vi "Panel.vi"(11 "Dashboard Panel in":refnum<class "Dashboard Panel.lvclass">) -> ()   [LabVIEW 2020, in "SB App.lvlib" / "Dashboard Panel.lvclass"]
uses:
  Dashboard Panel.lvclass
  C:/Program Files (x86)/National Instruments/LabVIEW 2020/vi.lib/IlluminatedG/IG OOPanel/OOPanel/Panel/Panel.lvclass
  Sort Type.ctl
  <vilib>/IlluminatedG/IG OOPanel/OOPanel/Panel/Basic UI State.ctl
  Dashboard Panel.lvclass/Dashboard Panel.ctl
  Team Dashboard Panel/Team Dashboard Panel.lvclass
  C:/Program Files (x86)/National Instruments/LabVIEW 2020/vi.lib/IlluminatedG/IG OOPanel/OOPanel/ArrayPanel/ArrayPanel.lvclass
  Active Sort.vi
  Killed Sort.vi
  Attacked Sort.vi
  Collisions Sort.vi
  Replicated Sort.vi
  <vilib>/IlluminatedG/IG OOPanel/OOPanel/ArrayManager/ArrayManager.lvclass
  SquareBattle/Team/Team.lvclass
  <vilib>/IlluminatedG/IG OOPanel/OOPanel/Panel/Panel.lvclass
  <vilib>/IlluminatedG/IG OOPanel/OOPanel/OOPanel.lvlib
panel:
  in  "Sort":T1
  out "Round":u32
  in  "Stop":bool
  in  "Step":bool
  in  "Start":bool
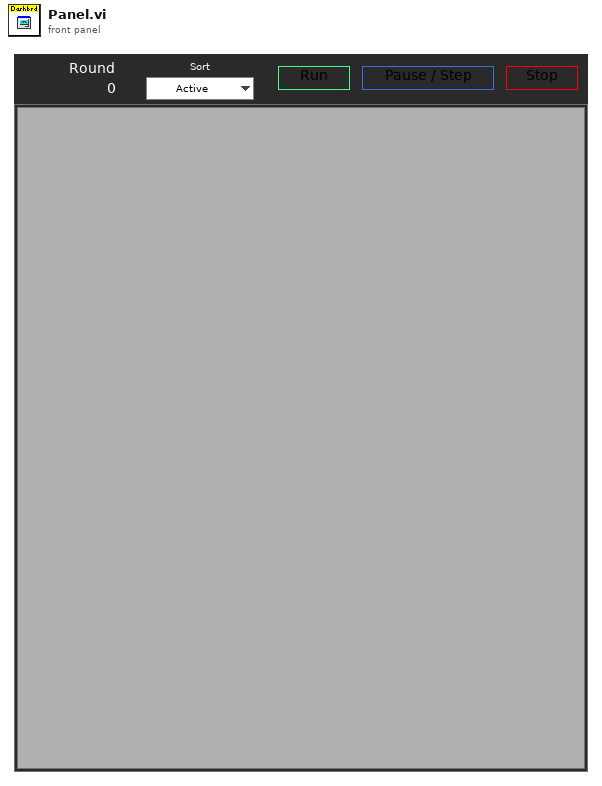
[diagram p1: front panel]
types:
  T1 = typedef "SB App.lvlib/Dashboard Panel.lvclass/Sort Type.ctl" = enum16{"Active", "Kills", "Attacked", "Collisions", "Replications"}
  T2 = typedef "OOPanel.lvlib/Panel.lvclass/Basic UI State.ctl" = enum16{"Init", "Run", "Close"}
  T3 = enum8{"Enabled", "Disabled", "Disabled and Grayed Out"}
  T4 = typedef "SB App.lvlib/Dashboard Panel.lvclass/Incoming Events.ctl" = cluster{"Round":refnum<user-event>, "Teams":refnum<user-event>, "Team Stats":refnum<user-event>}
  T5 = typedef "OOPanel.lvlib/Panel.lvclass/Panel Events.ctl" = cluster{"Visbility":refnum<user-event>, "Close":refnum<user-event>}
  T6 = typedef "SB App.lvlib/Team Status Data.ctl" = cluster{"Team Stats":T7, "Team State":T8}
  T7 = typedef "SquareBattle.lvlib/Team Stats.ctl" = cluster{"Active":i32, "Generated":i32, "Kills":i32, "Eliminated":i32, "Collided":i32}
  T8 = typedef "SquareBattle.lvlib/Team State.ctl" = enum16{"Active", "Defeated", "Won"}
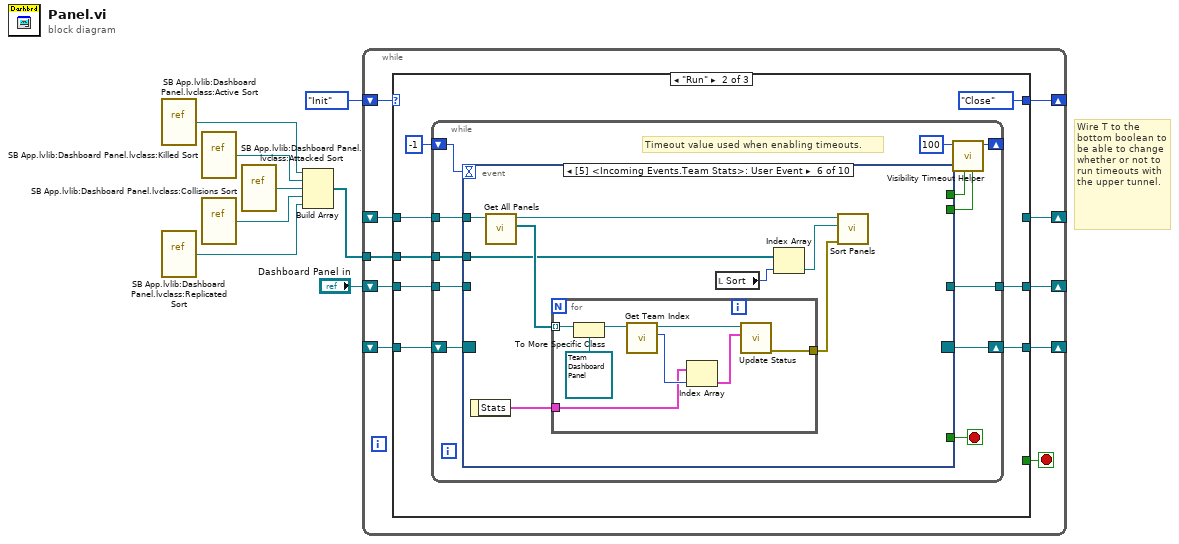
[diagram p0: block diagram]
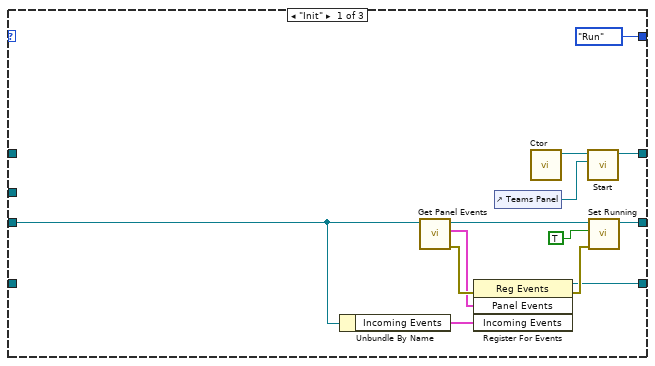
[diagram p2: hidden frame]
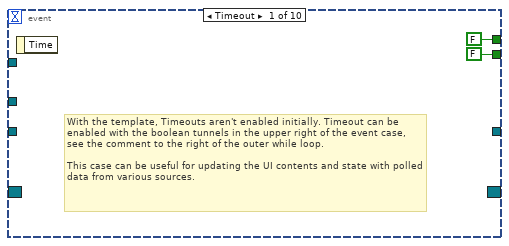
[diagram p3: hidden frame]
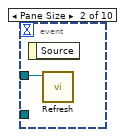
[diagram p4: hidden frame]
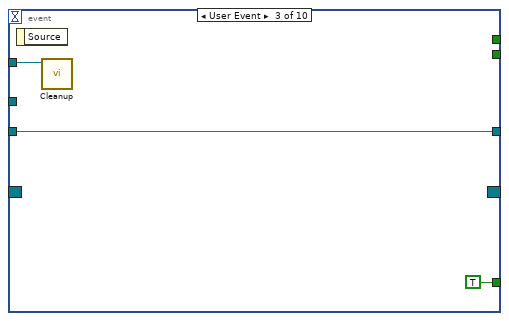
[diagram p5: hidden frame]
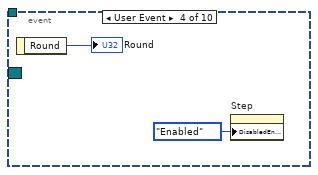
[diagram p6: hidden frame]
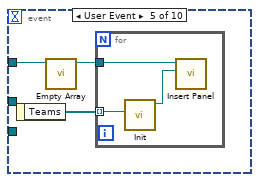
[diagram p7: hidden frame]
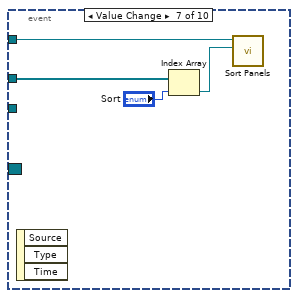
[diagram p8: hidden frame]
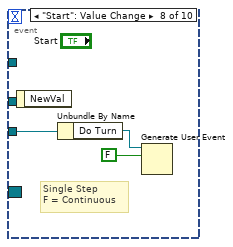
[diagram p9: hidden frame]
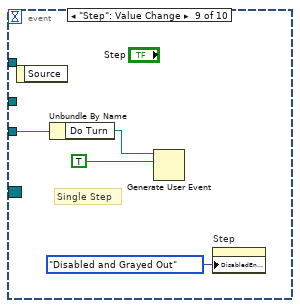
[diagram p10: hidden frame]
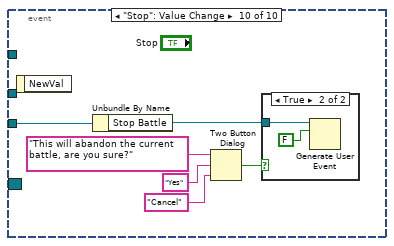
[diagram p11: hidden frame]
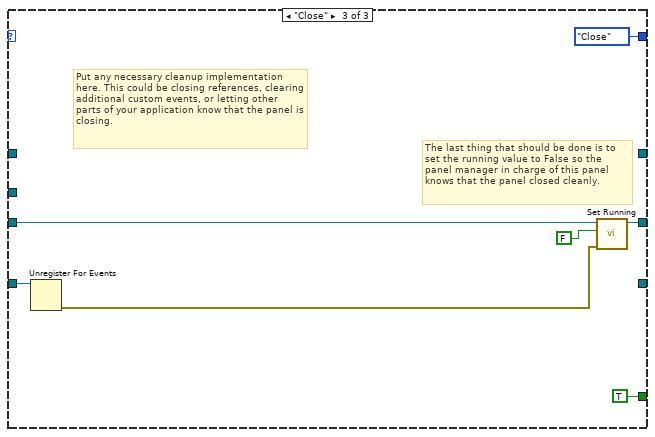
[diagram p13: hidden frame]
diagram:
  # "Wire T to the bottom boolean to be able to change whether or not to run timeouts with the upper tunnel."
  n1 = vi-ref "SB App.lvlib:Dashboard Panel.lvclass:Active Sort.vi"() -> (w6:refnum<vi>)
  n2 = vi-ref "SB App.lvlib:Dashboard Panel.lvclass:Replicated Sort.vi"() -> (w2:refnum<vi>)
  n3 = vi-ref "SB App.lvlib:Dashboard Panel.lvclass:Killed Sort.vi"() -> (w5:refnum<vi>)
  n4 = vi-ref "SB App.lvlib:Dashboard Panel.lvclass:Collisions Sort.vi"() -> (w3:refnum<vi>)
  n5 = vi-ref "SB App.lvlib:Dashboard Panel.lvclass:Attacked Sort.vi"() -> (w4:refnum<vi>)
  n6 = Build Array(w6, w5, w4, w3, w2) -> (w1:refnum<vi>[])
  n7 = while {
    shift-right: [w17] -> _
    shift-left: _ -> [w18]
    shift-right: [w15] -> _
    shift-left: Basic_UI_State."Init" ("Basic UI State") -> [w16]
    shift-right: [w13] -> _
    shift-left: "Dashboard Panel in" -> [w12]
    shift-right: [w11] -> _
    shift-left: _ -> [w10]
    tunnel: w1 -> [w9]
    stop <- w14 stop-if-true
    n8 = case shown="\"Run\"" w16 {
      tunnel: w18 -> [_ w39 w103]
      tunnel: [w25 w37 _] -> w17
      tunnel: [Basic_UI_State."Run" ("Basic UI State") Basic_UI_State."Close" ("Basic UI State") Basic_UI_State."Close" ("Basic UI State")] -> w15
      tunnel: [_ _ TRUE] -> w14
      tunnel: [w24 w34 w101] -> w13
      tunnel: w12 -> [w23 w35 w102]
      tunnel: [w19 _ _] -> w11
      tunnel: w10 -> [_ w33 _]
      tunnel: w9 -> [_ w32 _]
      frame "Init" {
        n9 = Unbundle By Name(w23) -> ("Incoming Events"=w22:T4)
        n10 = call <vilib>:"Get Panel Events.vi"("Panel in"=w23) -> ("error out"=w31:errorcluster, "Panel Events"=w27:T5, "Panel out"=w28:refnum<class "Dashboard Panel.lvclass">)  [unwired: 8 in]
        n11 = register-events(error in=w31, w27, w22) -> (reference out=w25:refnum<event-registration>, error out=w29:errorcluster)  [unwired: 1 in]
        n12 = control-ref of="Teams Panel"() -> (w20:refnum<vi>)
        n13 = call <vilib>:"Ctor.vi"() -> ("PanelArray"=w21:refnum<class "ArrayManager.lvclass">)  [unwired: 10 in, 1 out]
        n14 = call <vilib>:"Start.vi"("Container"=w20, "ArrayManager in"=w21) -> ("ArrayManager out"=w19:refnum<class "ArrayManager.lvclass">)  [unwired: 8 in, 1 out]
        n15 = call <vilib>:"Set Running.vi"("error in (no error)"=w29, "Running"=TRUE, "Panel in"=w28) -> ("Panel out"=w24:refnum<class "Dashboard Panel.lvclass">)  [unwired: 7 in, 1 out]
      }
      frame "Run" {
        n16 = while {
          shift-right: [w47] -> w37
          shift-left: w39 -> [w48]
          shift-right: [w50] -> _
          shift-left: -1 ("Timeout") -> [w49]
          tunnel: w35 -> [w43]
          tunnel: [w42] -> w34
          tunnel: w33 -> [w41]
          tunnel: w32 -> [w40]
          stop <- w44 stop-if-true
          # "Timeout value used when enabling timeouts."
          n17 = event shown="[5] <Incoming Events.Team Stats>: User Event" {
            selector: w48 -> [_ _ _ _ _ _ _ _ _ _]
            dyn-events: [_ _ _ _ _ _ _ _ _ _] -> w47
            timeout: w49 -> [_ _ _ _ _ _ _ _ _ _]
            tunnel: [FALSE _ _ _ _ _ _ _ _ _] -> w46
            tunnel: [FALSE _ _ _ _ _ _ _ _ _] -> w45
            tunnel: [_ _ TRUE _ _ _ _ _ _ _] -> w44
            tunnel: w43 -> [_ _ w56 _ _ _ _ w88 w92 w94]
            tunnel: [_ _ w56 _ _ _ _ _ _ _] -> w42
            tunnel: w41 -> [_ w54 w55 _ w62 w73 w83 _ _ _]
            tunnel: w40 -> [_ _ _ _ _ w68 w84 _ _ _]
            event Timeout {
              # "With the template, Timeouts aren't enabled initially. Timeout can be enabled with the boolean tunnels in the upper right of the event case, see the comment to the right of the outer while loop.\n\nThis case can be useful for updating the UI contents and state with polled data from various sources."
              n18 = event-data() -> ()  [unwired: 1 in, 1 out]
            }
            event Pane Size {
              n19 = event-data() -> ()  [unwired: 1 in, 1 out]
              n20 = call <vilib>:"Refresh.vi"("ArrayManager in"=w54) -> ()  [unwired: 9 in, 2 out]
            }
            event User Event {
              n21 = event-data() -> ()  [unwired: 1 in, 1 out]
              n22 = call <vilib>:"Cleanup.vi"("PanelArray in"=w55) -> ()  [unwired: 10 in, 1 out]
            }
            event User Event {
              n23 = event-data() -> ("Round"=→"Round":u32)  [unwired: 1 in]
              n24 = property on="Step" class="Bool"("DisabledEnum"=T3."Enabled" ("Disabled")) -> ()  [unwired: 2 in, 2 out]
            }
            event User Event {
              n25 = event-data() -> ("Teams"=w60:refnum<class "Team.lvclass">[])  [unwired: 1 in]
              n26 = call <vilib>:"Empty Array.vi"("ArrayManager in"=w62) -> ("ArrayManager out"=w61:refnum<class "ArrayManager.lvclass">)  [unwired: 9 in, 1 out]
              n27 = for {
                tunnel: w61 -> [w64]
                tunnel: w60 -> [w65] mode=indexing
                n28 = call "Init.vi"("Team"=w65) -> ("Team Dashboard Panel out"=w63:refnum<class "Team Dashboard Panel.lvclass">)  [unwired: 9 in, 1 out]
                n29 = call <vilib>:"Insert Panel.vi"("Panel/Type"=w63, "PanelArray in"=w64) -> ()  [unwired: 7 in, 3 out]
              }
            }
            event User Event {
              n30 = event-data() -> ("Stats"=w71:T6[])  [unwired: 1 in]
              n31 = call <vilib>:"Get All Panels.vi"("PanelArray in"=w73) -> ("Panels"=w72:refnum<class "ArrayPanel.lvclass">[], "PanelArray out"=w70:refnum<class "ArrayManager.lvclass">)  [unwired: 8 in, 1 out]
              n32 = for {
                tunnel: w72 -> [w81] mode=indexing
                tunnel: w71 -> [w75]
                tunnel: [w79] -> w69
                n33 = To More Specific Class(target class=refnum<class "Team Dashboard Panel.lvclass"> refnum ("SB App.lvlib:Team Dashboard Panel.lvclass"), reference=w81) -> (specific class reference=w78:refnum<class "Team Dashboard Panel.lvclass">)  [unwired: 1 in, 1 out]
                n34 = call "Get Team Index.vi"("Team Dashboard Panel in"=w78) -> ("Team Index"=w76:i32, "Team Dashboard Panel out"=w77:refnum<class "Team Dashboard Panel.lvclass">)  [unwired: 8 in, 1 out]
                n35 = Index Array(array=w75, index=w76) -> (element=w74:T6)
                n36 = call "Update Status.vi"("Team Status"=w74, "Team Dashboard Panel in"=w77) -> ("error out"=w79:errorcluster)  [unwired: 8 in, 1 out]
              }
              n37 = local read "Sort"() -> (w66:T1)
              n38 = Index Array(array=w68, index=w66) -> (element=w67:refnum<vi>)
              n39 = call <vilib>:"Sort Panels.vi"("error in (no error)"=w69, "Sort VI"=w67, "ArrayManager in"=w70) -> ()  [unwired: 7 in, 2 out]
            }
            event Value Change {
              n40 = event-data() -> ()  [unwired: 1 in, 3 out]
              n41 = Index Array(array=w84, index="Sort") -> (element=w85:refnum<vi>)
              n42 = call <vilib>:"Sort Panels.vi"("Sort VI"=w85, "ArrayManager in"=w83) -> ()  [unwired: 8 in, 2 out]
            }
            event "Start": Value Change {
              # "Single Step\nF = Continuous"
              n43 = event-data() -> ()  [unwired: 1 in, 1 out]
              n44 = Unbundle By Name(w88) -> ("Do Turn"=w87:refnum<user-event>)
              n45 = Generate User Event(user event=w87, event data cluster=FALSE ("event data")) -> ()  [unwired: 2 in, 2 out]
            }
            event "Step": Value Change {
              # "Single Step"
              n46 = event-data() -> ()  [unwired: 1 in, 1 out]
              n47 = Unbundle By Name(w92) -> ("Do Turn"=w91:refnum<user-event>)
              n48 = Generate User Event(user event=w91, event data cluster=TRUE ("event data")) -> ()  [unwired: 2 in, 2 out]
              n49 = property on="Step" class="Bool"("DisabledEnum"=T3."Disabled and Grayed Out" ("Disabled")) -> ()  [unwired: 2 in, 2 out]
            }
            event "Stop": Value Change {
              n50 = event-data() -> ()  [unwired: 1 in, 1 out]
              n51 = Unbundle By Name(w94) -> ("Stop Battle"=w93:refnum<user-event>)
              n52 = Two Button Dialog(message="This will abandon the current battle, are you sure?", 1:"Cancel" ("T button name (\"OK\")"), 2:"Yes" ("T button name (\"OK\")")) -> (T button?=w95:bool)
              n53 = case shown="True" w95 {
                tunnel: w93 -> [_ w100]
                frame False {
                }
                frame True {
                  n54 = Generate User Event(user event=w100, event data cluster=FALSE) -> ()  [unwired: 2 in, 2 out]
                }
              }
            }
          }
          n55 = call <vilib>:"Visibility Timeout Helper.vi"("Update?"=w45, "Use Timeout?"=w46, "Visible Timeout mS"=100) -> ("Timeout"=w50:i32)  [unwired: 8 in]
        }
      }
      frame "Close" {
        # "Put any necessary cleanup implementation here. This could be closing references, clearing additional custom events, or letting other parts of your application know that the panel is closing."
        # "The last thing that should be done is to set the running value to False so the panel manager in charge of this panel knows that the panel closed cleanly."
        n56 = Unregister For Events(event registration refnum=w103) -> (error out=w105:errorcluster)  [unwired: 1 in]
        n57 = call <vilib>:"Set Running.vi"("error in (no error)"=w105, "Running"=FALSE, "Panel in"=w102) -> ("Panel out"=w101:refnum<class "Dashboard Panel.lvclass">)  [unwired: 7 in, 1 out]
      }
    }
  }
